vi "User.File.Write.vi"(8 "error in (no error)":errorcluster) -> (0 "error out":errorcluster)   [LabVIEW 2016]
uses:
  User.Info.ctl
  User.Level.ctl
  User.Global.vi
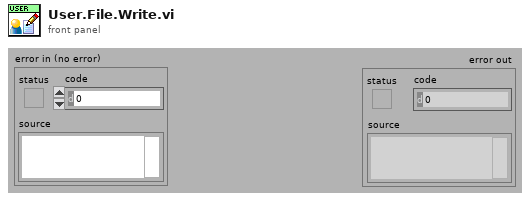
[diagram p1: front panel]
types:
  T1 = typedef "User.Info.ctl" = cluster{"ID":i32, "Name":string, "Pass":string, "Level":T2, "Del":bool}
  T2 = typedef "User.Level.ctl" = enum16{"-", "Operator", "Technician", "Administrator"}
  T3 = cluster{"Users":T1[], "Temp":string, "TS":timestamp, "Operator":string, "User":string, "Duration":dbl}
  T4 = cluster{"f":u8[], "u":u8[], "c":u8[][], "k":u8[][], "u2":u8[][]}
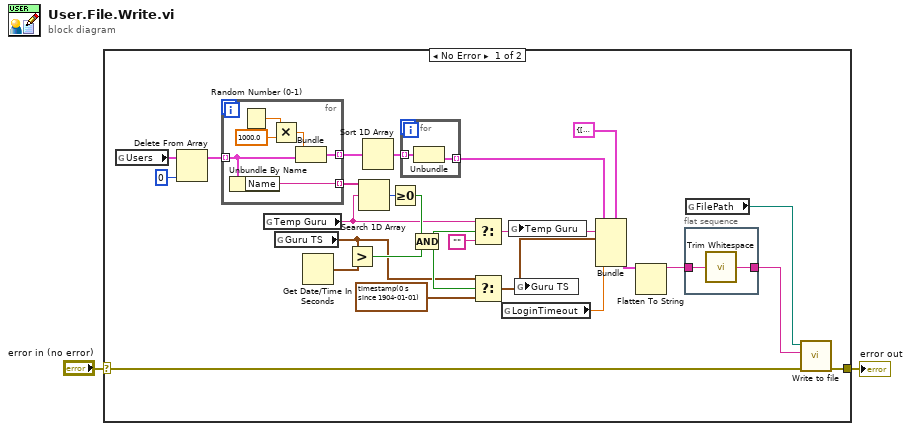
[diagram p0: block diagram]
diagram:
  n1 = case shown="No Error" "error in (no error)" {
    selector: "error in (no error)" -> [w27 w169]
    tunnel: [w28 w169] -> w1
    frame No Error {
      n2 = global read "User.Global.vi" "Users"() -> (w26:T1[])
      n3 = Delete From Array(array=w26, index=0) -> (array with subset deleted=w11:T1[])  [unwired: 1 in, 1 out]
      n4 = for {
        tunnel: w11 -> [w32] mode=indexing
        tunnel: [w33] -> w23 mode=indexing
        tunnel: [w31] -> w21 mode=indexing
        n5 = Unbundle By Name(w32) -> ("Name"=w31:string)
        n6 = Random Number (0-1)() -> (number: 0 to 1=w35:dbl)
        n7 = Multiply(x=w35, y=1000.0) -> (x*y=w34:dbl)
        n8 = Bundle(w34, "User Info"=w32) -> (w33:cluster{dbl, "User Info":T1})  [unwired: 1 in]
      }
      n9 = global read "User.Global.vi" "Temp Guru"() -> (w13:string)
      n10 = global read "User.Global.vi" "Guru TS"() -> (w12:timestamp)
      n11 = Get Date/Time In Seconds() -> (seconds since 1Jan1904=w18:timestamp)
      n12 = Greater?(x=w12, y=w18) -> (0:w15:bool)
      n13 = Search 1D Array(1D array=w21, element=w13) -> (index of element=w17:i32)  [unwired: 1 in]
      n14 = Sort 1D Array(array=w23) -> (sorted array=w22:cluster{dbl, "User Info":T1}[])
      n15 = Greater Or Equal To 0?(x=w17) -> (x >= 0?=w16:bool)
      n16 = for {
        tunnel: w22 -> [w30] mode=indexing
        tunnel: [w29] -> w10 mode=indexing
        n17 = Unbundle(w30) -> ("User Info"=w29:T1)  [unwired: 1 out]
      }
      n18 = Compound Arithmetic op=AND(w16, w15) -> (w14:bool)
      n19 = Select(t=w13, s=w14, f="") -> (s? t:f=w9:string)
      n20 = Select(t=w12, s=w14, f=timestamp(0 s since 1904-01-01)) -> (s? t:f=w5:timestamp)
      n21 = global read "User.Global.vi" "LoginTimeout"() -> (w4:dbl)
      n22 = global write "User.Global.vi" "Temp Guru"(w9) -> ()
      n23 = global write "User.Global.vi" "Guru TS"(w5) -> ()
      n24 = Bundle(cluster=T3 {"Users"=[], "Temp"="", "TS"=timestamp(0 s since 1904-01-01), "Operator"="Service", "User"="Admin", "Duration"=5.0}, "Users"=w10, "Temp"=w9, "TS"=w5, "Duration"=w4) -> (w8:T3)  [unwired: 2 in]
      n25 = Flatten To String(anything=w8) -> (data string=w24:string)  [unwired: 3 in, 2 out]
      n26 = flat-sequence {
        tunnel: [w37] -> w25
        tunnel: w24 -> [w38]
        frame #0 {
          n27 = disable-structure shown="Enabled" {
            disable-tunnel: w38 -> [w42 _]
            disable-tunnel: [w40 _] -> w37
            frame Enabled {
              w49 = 16 ("length (rest)")
              n28 = String To Byte Array(string=w42) -> (unsigned byte array=w51:u8[])
              n29 = Array Size(array=w51) -> (size(s)=w52:i32)
              n30 = Divide(x=w52, y=w49) -> (x/y=w50:dbl)
              n31 = Round Toward +Infinity(x=w50) -> (ceil(x): smallest int >= x=w48:dbl)
              n32 = Unbundle By Name(T4 {"f"=[99, 124, 119, 123, 242, 107, 111, 197, 48, 1, 103, 43, 254, 215, 171, 118, 202, 130, 201, 125, 250, 89, 71, 240, 173, 212, 162, 175, 156, 164, 114, 192, 183, 253, 147, 38, 54, 63, 247, 204, 52, 165, 229, 241, 113, 216, 49, 21, 4, 199, 35, 195, 24, 150, 5, 154, 7, 18, 128, 226, 235, 39, 178, 117, 9, 131, 44, 26, 27, 110, 90, 160, 82, 59, 214, 179, 41, 227, 47, 132, 83, 209, 0, 237, 32, 252, 177, 91, 106, 203, 190, 57, 74, 76, 88, 207, 208, 239, 170, 251, 67, 77, 51, 133, 69, 249, 2, 127, 80, 60, 159, 168, 81, 163, 64, 143, 146, 157, 56, 245, 188, 182, 218, 33, 16, 255, 243, 210, 205, 12, 19, 236, 95, 151, 68, 23, 196, 167, 126, 61, 100, 93, 25, 115, 96, 129, 79, 220, 34, 42, 144, 136, 70, 238, 184, 20, 222, 94, 11, 219, 224, 50, 58, 10, 73, 6, 36, 92, 194, 211, 172, 98, 145, 149, 228, 121, 231, 200, 55, 109, 141, 213, 78, 169, 108, 86, 244, 234, 101, 122, 174, 8, 186, 120, 37, 46, 28, 166, 180, 198, 232, 221, 116, 31, 75, 189, 139, 138, 112, 62, 181, 102, 72, 3, 246, 14, 97, 53, 87, 185, 134, 193, 29, 158, 225, 248, 152, 17, 105, 217, 142, 148, 155, 30, 135, 233, 206, 85, 40, 223, 140, 161, 137, 13, 191, 230, 66, 104, 65, 153, 45, 15, 176, 84, 187, 22], "u"=[82, 9, 106, 213, 48, 54, 165, 56, 191, 64, 163, 158, 129, 243, 215, 251, 124, 227, 57, 130, 155, 47, 255, 135, 52, 142, 67, 68, 196, 222, 233, 203, 84, 123, 148, 50, 166, 194, 35, 61, 238, 76, 149, 11, 66, 250, 195, 78, 8, 46, 161, 102, 40, 217, 36, 178, 118, 91, 162, 73, 109, 139, 209, 37, 114, 248, 246, 100, 134, 104, 152, 22, 212, 164, 92, 204, 93, 101, 182, 146, 108, 112, 72, 80, 253, 237, 185, 218, 94, 21, 70, 87, 167, 141, 157, 132, 144, 216, 171, 0, 140, 188, 211, 10, 247, 228, 88, 5, 184, 179, 69, 6, 208, 44, 30, 143, 202, 63, 15, 2, 193, 175, 189, 3, 1, 19, 138, 107, 58, 145, 17, 65, 79, 103, 220, 234, 151, 242, 207, 206, 240, 180, 230, 115, 150, 172, 116, 34, 231, 173, 53, 133, 226, 249, 55, 232, 28, 117, 223, 110, 71, 241, 26, 113, 29, 41, 197, 137, 111, 183, 98, 14, 170, 24, 190, 27, 252, 86, 62, 75, 198, 210, 121, 32, 154, 219, 192, 254, 120, 205, 90, 244, 31, 221, 168, 51, 136, 7, 199, 49, 177, 18, 16, 89, 39, 128, 236, 95, 96, 81, 127, 169, 25, 181, 74, 13, 45, 229, 122, 159, 147, 201, 156, 239, 160, 224, 59, 77, 174, 42, 245, 176, 200, 235, 187, 60, 131, 83, 153, 97, 23, 43, 4, 126, 186, 119, 214, 38, 225, 105, 20, 99, 85, 33, 12, 125], "c"=[[90, 1, 69, 10], [61, 7, 207, 135], [244, 76, 178, 236], [74, 228, 164, 36], [49, 56, 198, 20], [216, 46, 208, 179], [133, 132, 236, 77], [207, 242, 209, 46], [50, 72, 115, 220], [12, 63, 9, 147], [44, 98, 98, 95], [207, 96, 72, 105], [186, 6, 247, 158], [234, 102, 163, 111], [137, 187, 229, 222], [227, 144, 179, 113], [230, 26, 138, 86], [182, 57, 254, 13], [198, 4, 193, 48], [70, 219, 173, 183], [210, 107, 84, 143], [12, 124, 41, 57], [63, 130, 27, 211], [37, 148, 114, 65], [79, 143, 35, 12], [100, 82, 170, 130], [202, 120, 232, 9], [121, 89, 182, 100], [208, 43, 215, 176], [67, 243, 10, 53], [91, 208, 177, 81], [239, 236, 154, 72], [196, 193, 96, 186], [180, 121, 125, 50], [137, 139, 226, 60], [34, 137, 7, 53], [158, 147, 133, 111], [135, 50, 106, 143], [239, 169, 204, 99], [102, 103, 120, 116], [120, 4, 246, 41], [42, 234, 248, 93], [14, 185, 136, 179], [205, 32, 203, 86], [45, 47, 23, 92], [255, 54, 156, 166], [197, 67, 52, 62], [104, 222, 240, 199], [163, 27, 71, 148], [7, 197, 239, 1], [241, 143, 20, 21], [8, 99, 255, 104], [232, 163, 209, 25], [92, 45, 219, 50], [194, 134, 219, 63], [153, 81, 228, 210], [243, 13, 2, 164], [239, 102, 62, 24], [173, 162, 207, 39], [202, 229, 36, 87], [116, 202, 100, 247], [175, 32, 217, 150], [45, 224, 229, 39], [52, 243, 43, 245]], "k"=[[2, 3, 1, 1], [1, 2, 3, 1], [1, 1, 2, 3], [3, 1, 1, 2]], "u2"=[[14, 11, 13, 9], [9, 14, 11, 13], [13, 9, 14, 11], [11, 13, 9, 14]]} ("Cipher Keys")) -> ("c"=w46:u8[][], "f"=w45:u8[], "k"=w47:u8[][])
              n33 = Reshape Array(w51, w48, w49) -> (w44:u8[][])
              n34 = for {
                tunnel: w44 -> [w58] mode=indexing
                tunnel: w47 -> [w77]
                tunnel: w46 -> [w71]
                tunnel: [w66] -> w41 mode=indexing
                tunnel: w45 -> [w65]
                shift-right: [w54] -> _
                shift-left: u8[] [0, 0, 0, 0, 0, 0, 0, 0, 0, 0, 0, 0, 0, 0, 0, 0] ("initialized array") -> [w56]
                tunnel: TRUE ("Cipher Block Chaining (CBC)") -> [w55]
                w85 = 4 ("index")
                n35 = case shown="True" w55 {
                  tunnel: w58 -> [w86 w89]
                  tunnel: [w86 w88] -> w57
                  tunnel: w56 -> [_ w87]
                  frame False {
                  }
                  frame True {
                    n36 = Exclusive Or(1:w89, 2:w87) -> (0:w88:u8[])
                  }
                }
                n37 = Reshape Array(w57, w85, w85) -> (w81:u8[][])
                n38 = Array Subset(array=w71, index (row)=0, length (col)=4 ("length")) -> (w83:u8[][])  [unwired: 2 in]
                n39 = Transpose 2D Array ("state")(2D array=w81) -> (transposed array=w80:u8[][])
                n40 = Transpose 2D Array(2D array=w83) -> (transposed array=w79:u8[][])
                n41 = Exclusive Or ("add_round_key")(1:w79, 2:w80) -> (0:w76:u8[][])
                n42 = for {
                  N: 9 -> [_]
                  tunnel: w77 -> [w112]
                  shift-right: [w103] -> w75
                  shift-left: w76 -> [w107]
                  tunnel: w71 -> [w101]
                  tunnel: [w101] -> w63
                  tunnel: [w100] -> w64
                  tunnel: w65 -> [w100]
                  i -> [w106]
                  n43 = for "sub_bytes" {
                    tunnel: w100 -> [w165]
                    tunnel: w107 -> [w164] mode=indexing
                    tunnel: [w163] -> w113 mode=indexing
                    n44 = for {
                      tunnel: w165 -> [w168]
                      tunnel: w164 -> [w167] mode=indexing
                      tunnel: [w166] -> w163 mode=indexing
                      n45 = Index Array(array=w168, index=w167) -> (element=w166:u8)
                    }
                  }
                  n46 = for "shift_rows" {
                    tunnel: w113 -> [w162] mode=indexing
                    tunnel: [w160] -> w111 mode=indexing
                    i -> [w161]
                    n47 = Negate(x=w161) -> (-x=w159:i32)
                    n48 = Rotate 1D Array(1:w162, 2:w159) -> (0:w160:u8[])
                  }
                  n49 = Transpose 2D Array(2D array=w111) -> (transposed array=w110:u8[][])
                  n50 = for "mix_columns" {
                    tunnel: w112 -> [w116] mode=indexing
                    tunnel: w110 -> [w114]
                    tunnel: [w115] -> w104 mode=indexing
                    n51 = for {
                      tunnel: w116 -> [w120]
                      tunnel: [w118] -> w115 mode=indexing
                      tunnel: w114 -> [w117] mode=indexing
                      n52 = for {
                        tunnel: w120 -> [w122] mode=indexing
                        shift-right: [w133] -> w118
                        shift-left: u8 0 -> [w132]
                        tunnel: w117 -> [w123] mode=indexing
                        n53 = To Unsigned Word Integer(number=w123) -> (unsigned 16bit integer=w125:u16)
                        n54 = Number To Boolean Array(number=w122) -> (Boolean array=w126:bool[])
                        n55 = for {
                          N: 8 -> [_]
                          shift-right: [w151] -> w127
                          shift-left: u16 0 ("prod") -> [w152]
                          tunnel: w126 -> [w149] mode=indexing
                          tunnel: w125 -> [w148]
                          i -> [w150]
                          n56 = case shown="True" w149 {
                            tunnel: w150 -> [_ w155]
                            tunnel: w152 -> [w153 w158]
                            tunnel: [w153 w156] -> w151
                            tunnel: w148 -> [_ w154]
                            frame False {
                            }
                            frame True {
                              n57 = Logical Shift(y=w155, x=w154) -> (x << y=w157:u16)
                              n58 = Exclusive Or(1:w157, 2:w158) -> (0:w156:u16)
                            }
                          }
                        }
                        n59 = for {
                          N: 8 -> [_]
                          shift-right: [w136] -> w131
                          shift-left: w127 -> [w137]
                          tunnel: 283 ("mod_pol") -> [w134]
                          i -> [w140]
                          n60 = expression code="15-x"(w140) -> (w135:i32)
                          n61 = Number To Boolean Array(number=w137) -> (Boolean array=w139:bool[])
                          n62 = Index Array(array=w139, index=w135) -> (element=w138:bool)
                          n63 = case shown="True" w138 {
                            tunnel: w135 -> [_ w146]
                            tunnel: w137 -> [w141 w145]
                            tunnel: [w141 w143] -> w136
                            tunnel: w134 -> [_ w142]
                            frame False {
                            }
                            frame True {
                              n64 = expression code="x-8"(w146) -> (w147:i32)
                              n65 = Logical Shift(y=w147, x=w142) -> (x << y=w144:i32)
                              n66 = Exclusive Or(1:w144, 2:w145) -> (0:w143:i32)
                            }
                          }
                        }
                        n67 = To Unsigned Byte Integer(number=w131) -> (unsigned 8bit integer=w121:u8)
                        n68 = Exclusive Or(1:w132, 2:w121) -> (0:w133:u8)
                      }
                    }
                  }
                  n69 = expression code="4*(x+1)"(w106) -> (w105:i32)
                  n70 = Array Subset(array=w101, index (row)=w105, length (col)=4 ("length")) -> (w109:u8[][])  [unwired: 2 in]
                  n71 = Transpose 2D Array(2D array=w109) -> (transposed array=w102:u8[][])
                  n72 = Exclusive Or(1:w102, 2:w104) -> (0:w103:u8[][])
                }
                n73 = for "sub_bytes" {
                  tunnel: w64 -> [w96]
                  tunnel: w75 -> [w95] mode=indexing
                  tunnel: [w94] -> w74 mode=indexing
                  n74 = for {
                    tunnel: w96 -> [w99]
                    tunnel: w95 -> [w98] mode=indexing
                    tunnel: [w97] -> w94 mode=indexing
                    n75 = Index Array(array=w99, index=w98) -> (element=w97:u8)
                  }
                }
                n76 = Array Size(array=w63) -> (size(s)=w62:i32[])
                n77 = Index Array(array=w62, index=0) -> (element=w60:i32)
                n78 = expression code="x-4"(w60) -> (w59:i32)
                n79 = for "shift_rows" {
                  tunnel: w74 -> [w93] mode=indexing
                  tunnel: [w91] -> w70 mode=indexing
                  i -> [w92]
                  n80 = Negate(x=w92) -> (-x=w90:i32)
                  n81 = Rotate 1D Array(1:w93, 2:w90) -> (0:w91:u8[])
                }
                n82 = Array Subset(array=w63, index (row)=w59, length (col)=4 ("length")) -> (w73:u8[][])  [unwired: 2 in]
                n83 = Transpose 2D Array(2D array=w73) -> (transposed array=w69:u8[][])
                n84 = Exclusive Or(1:w69, 2:w70) -> (0:w68:u8[][])
                n85 = Reshape Array(w68, 16 ("dimension size")) -> (w54:u8[])
                n86 = Byte Array To String(unsigned byte array=w54) -> (string=w66:string)
              }
              n87 = Concatenate Strings(w41) -> (w40:string)
            }
            frame Disabled {
            }
          }
          n88 = call <vilib>:"Trim Whitespace.vi"("string"=w37) -> ()  [unwired: 1 in, 1 out]
        }
      }
      n89 = global read "User.Global.vi" "FilePath"() -> (w3:path)
      n90 = call "Write to file.vi"("error in"=w27, "addition"=w25, "file"=w3) -> ("error out"=w28:errorcluster)  [unwired: 8 in]
    }
    frame Error {
    }
  }
  "error out" <- w1
